vi "vetorcordist.vi"(9 "Parâmetros 2":T2={"Azul Max EV3 Cor"=17, "Azul Min EV3 Cor"=0, "Verde Max EV3 Cor"=6, "Verde Min EV3 Cor"=0, "Vermelho Max Ev3 Cor"=0, "Vermelho Min EV3 Cor"=0, "Chão EV3 Cor"=0.0, "Branco Max EV3 Cor"=0.0, "Branco Min EV3 Cor"=0.0, "Preto Max EV3 Cor"=0.0, "Preto Min EV3 Cor"=0.0, "Distância Tubulação"=0.0, "Distância Frontal"=0.0, "Amarelo Max EV3 Cor"=0.0, "Amarelo Min EV3 Cor"=0.0, "Distância Lateral"=0.0, "90°"=0.0, "180°"=0.0, "Seguidor de Linha"=0.0}, 11 "NXT/EV3 2":T1) -> (0 "dist perc":dbl, 3 "NXT/EV3 13":T1, 8 "cod cor":dbl format="%#_13g")   [LabVIEW 2016]
uses:
  <vilib>/NXT/Subs/LVHSConnector.ctl
  <vilib>/NXT/LegoClasses/BrickReference/BrickReference.lvclass
  <vilib>/NXT/Block Support/NXT_InputPort.ctl
  <vilib>/NXT/Block Support/NXT_OutputPort.ctl
  <vilib>/NXT/Dual Mode Library/Sensors/EV3_Gyro_Reset.vi
  <vilib>/NXT/Dual Mode Library/Motors/ResetMotor.vi
  <vilib>/NXT/Dual Mode Library/Sensors/EV3_Gyro_Angle.vi
  <vilib>/NXT/NXTIO Xnodes/NXTIONodeSubVIs/NXTStopMotors.vi
  <vilib>/NXT/Dual Mode Library/Motors/Rotation.vi
  <vilib>/NXT/NXTIO Xnodes/AddressXNode/NXTIOAddress.xnode
  <vilib>/NXT/NXTIO Xnodes/NXTIOXNode/NXTIO.xnode
panel:
  # "Sensor EV3 Cor"
  # "Sensor Ultrassônico"
  # "Sensor Giroscópio"
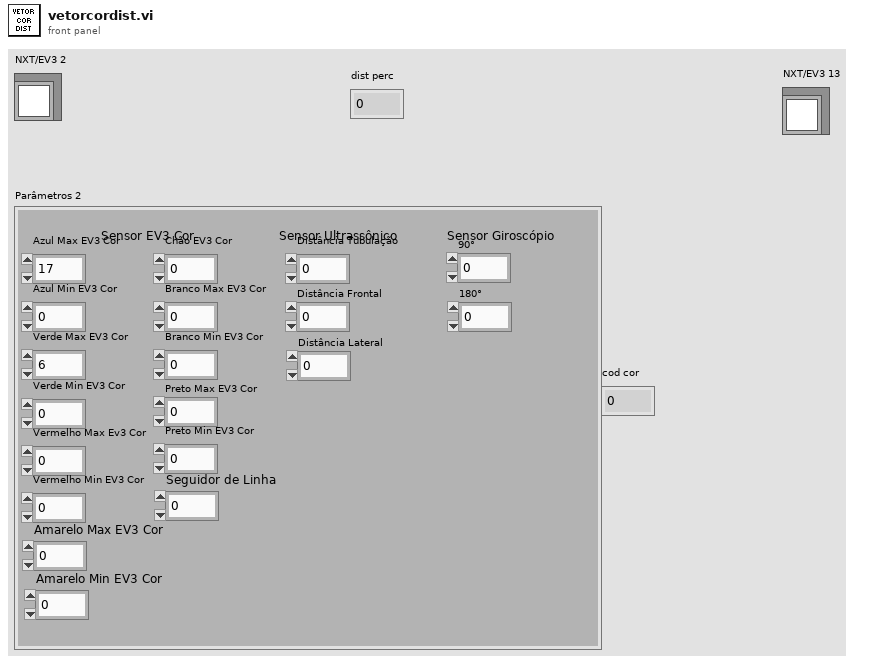
[diagram p1: front panel]
types:
  T1 = typedef "LVHSConnector.ctl" = refnum<class "BrickReference.lvclass">
  T2 = cluster{"Azul Max EV3 Cor":i32, "Azul Min EV3 Cor":i32, "Verde Max EV3 Cor":i32, "Verde Min EV3 Cor":i32, "Vermelho Max Ev3 Cor":i32, "Vermelho Min EV3 Cor":i32, "Chão EV3 Cor":sgl, "Branco Max EV3 Cor":sgl, "Branco Min EV3 Cor":sgl, "Preto Max EV3 Cor":sgl, "Preto Min EV3 Cor":sgl, "Distância Tubulação":sgl, "Distância Frontal":sgl, "Amarelo Max EV3 Cor":dbl, "Amarelo Min EV3 Cor":dbl, "Distância Lateral":sgl, "90°":sgl, "180°":sgl, "Seguidor de Linha":dbl}
  T3 = typedef "NXT_OutputPort.ctl" = u8
  T4 = typedef "NXT_InputPort.ctl" = u32
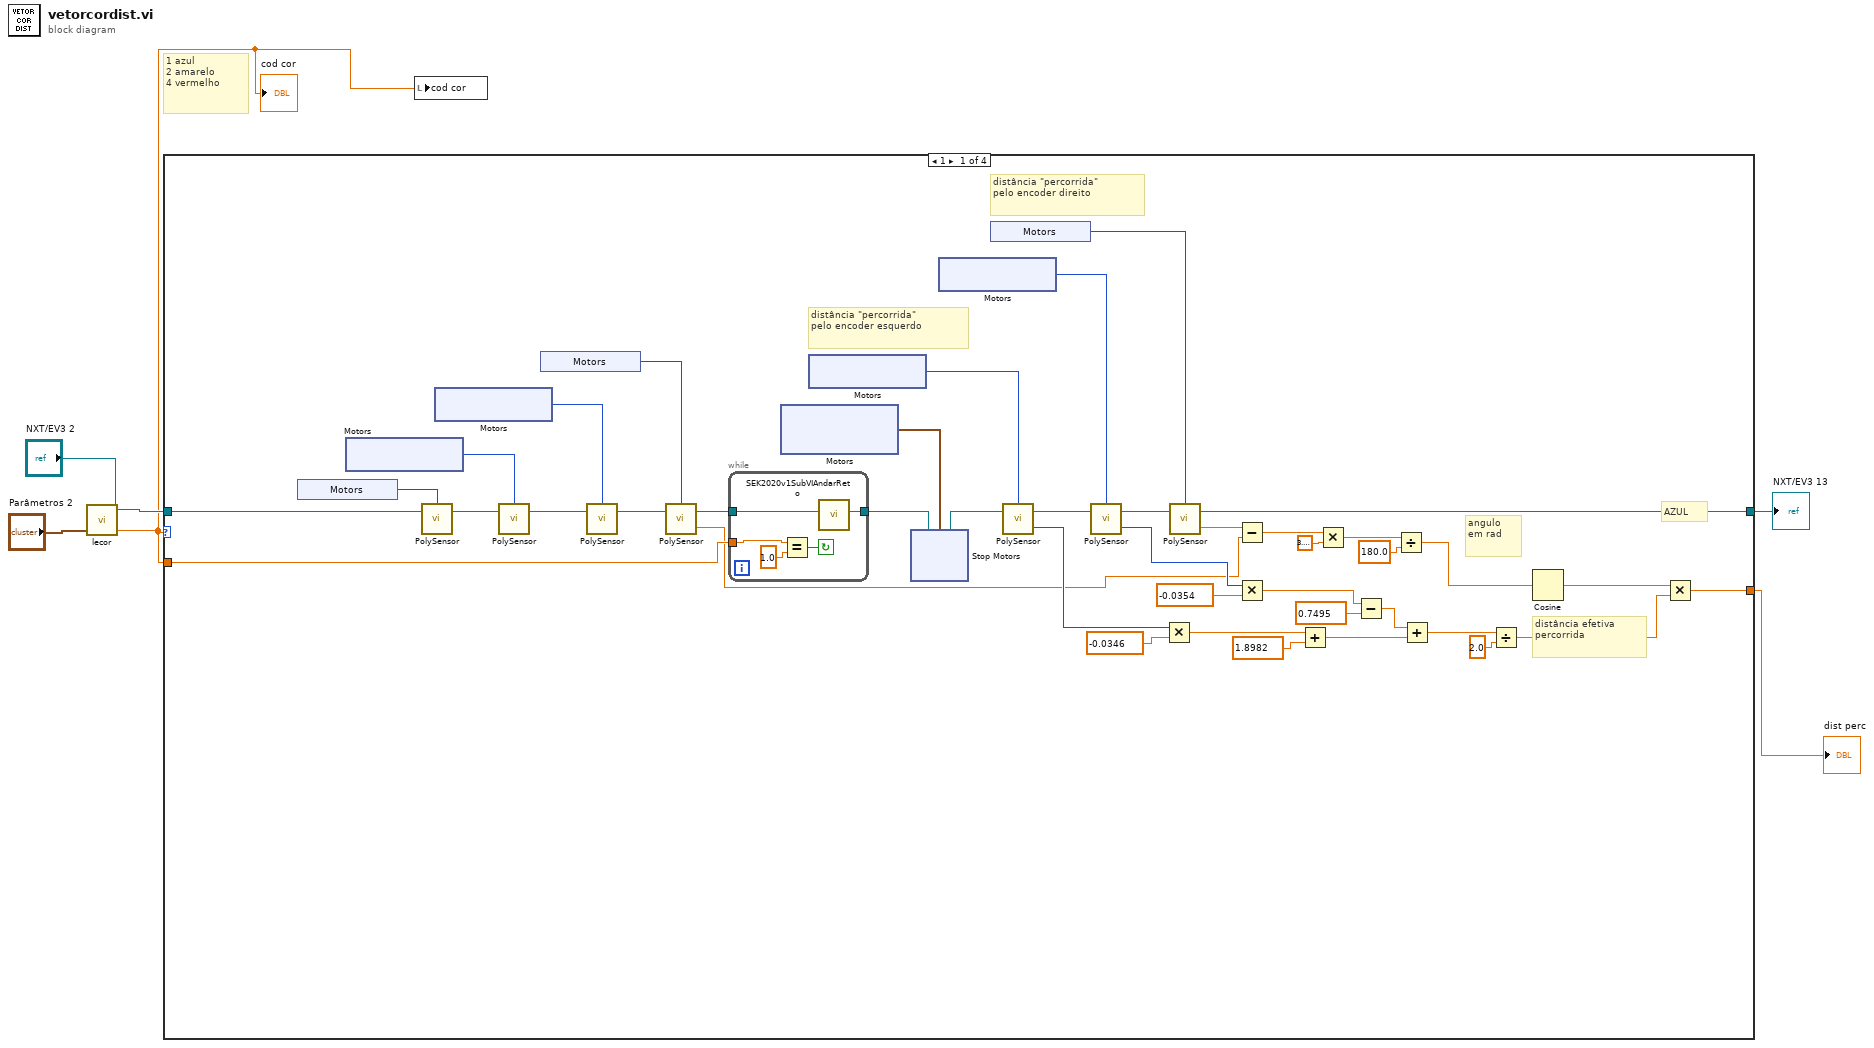
[diagram p0: block diagram]
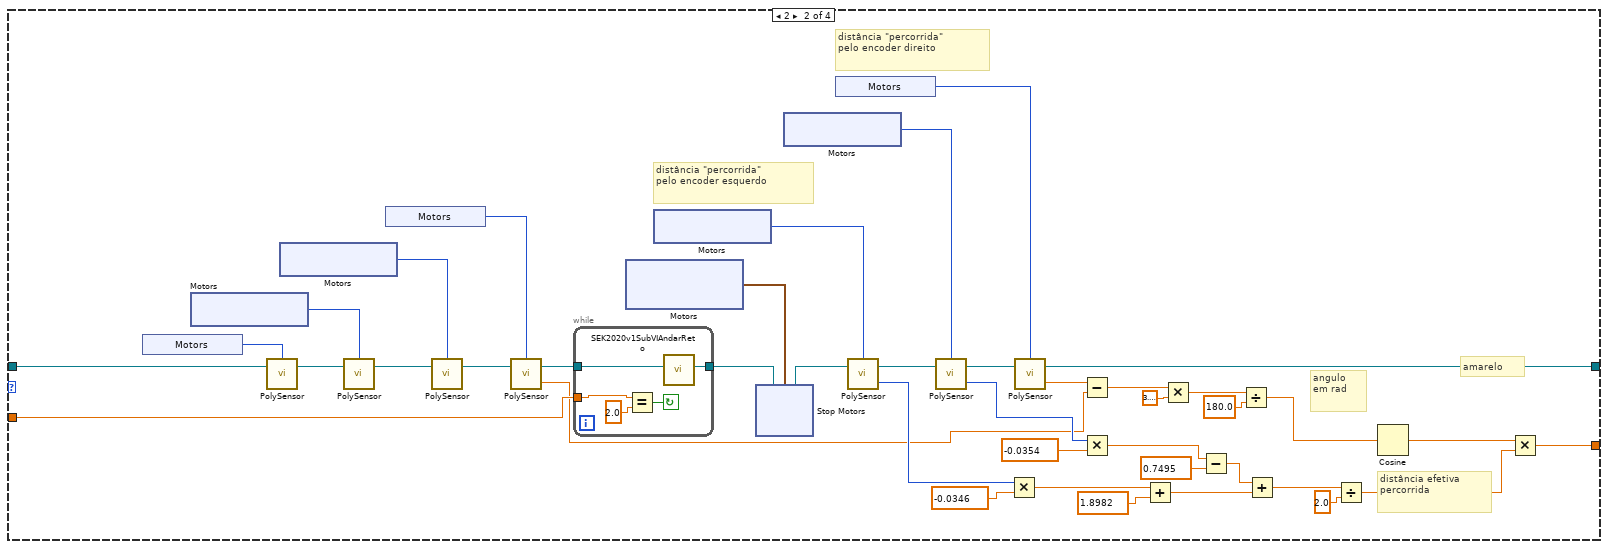
[diagram p2: hidden frame]
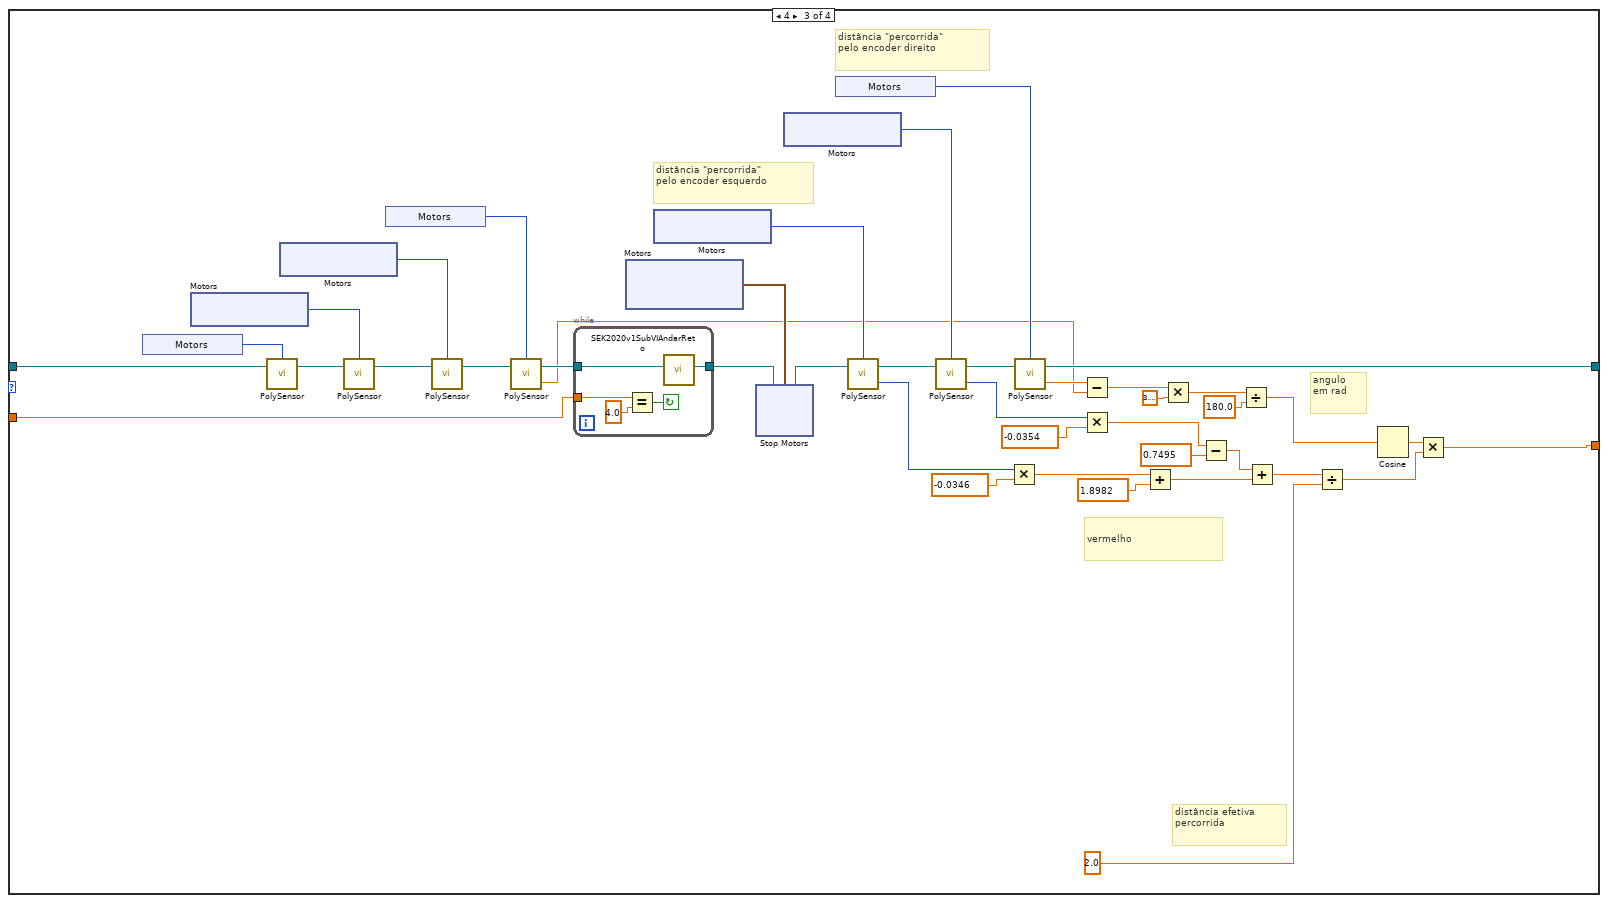
[diagram p3: hidden frame]
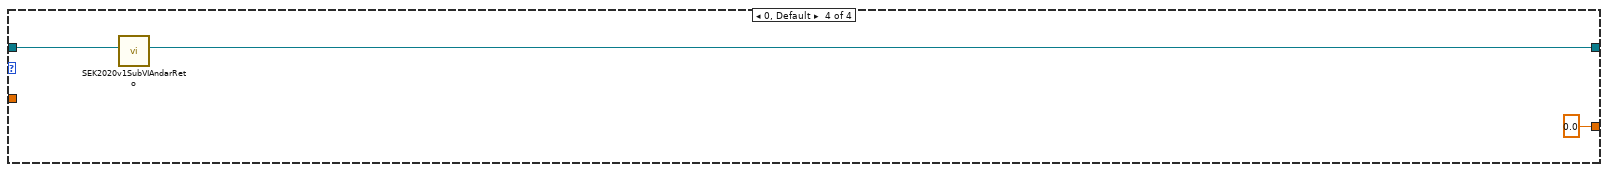
[diagram p4: hidden frame]
diagram:
  # "1 azul\n2 amarelo\n4 vermelho"
  n1 = call "lecor.vi"("Parâmetros 2"="Parâmetros 2", "NXT/EV3"="NXT/EV3 2") -> ("cor"=w1:dbl, "NXT/EV3 2"=w4:T1)  [unwired: 2 in]
  "cod cor" <- w1
  n2 = case shown="1" w1 {
    tunnel: w4 -> [w12 w71 w130 w186]
    tunnel: [w47 w106 w165 w185] -> w3
    tunnel: [w46 w105 w164 0.0] -> w2
    tunnel: w1 -> [w11 w70 w129 _]
    frame 1 {
      # "AZUL"
      # "angulo \nem rad"
      # "distância efetiva\npercorrida"
      # "distância \"percorrida\" \npelo encoder direito"
      # "distância \"percorrida\" \npelo encoder esquerdo"
      n3 = xnode "Motors"() -> ("Sensor"=w16:T4)
      n4 = xnode "Motors"() -> ("Motor"=w18:T3)
      n5 = call-poly <vilib>:"PolySensor.vi"("NXT/EV3"=w12, "Port (Port 1)"=w16) -> ("NXT/EV3"=w15:T1)  [unwired: 2 in]
      n6 = xnode "Motors"() -> ("Motor"=w13:T3)
      n7 = call-poly <vilib>:"PolySensor.vi"("NXT/EV3"=w15, "Port (All Ports)"=w18) -> ("NXT/EV3"=w17:T1)  [unwired: 2 in]
      n8 = xnode "Motors"() -> ("Sensor"=w10:T4)
      n9 = call-poly <vilib>:"PolySensor.vi"("NXT/EV3"=w17, "Port (All Ports)"=w13) -> ("NXT/EV3"=w9:T1)  [unwired: 2 in]
      n10 = call-poly <vilib>:"PolySensor.vi"("NXT/EV3"=w9, "Port (Port 1)"=w10) -> ("Degrees"=w7:sgl, "NXT/EV3"=w8:T1)  [unwired: 1 in]
      n11 = while {
        tunnel: [w53] -> w14
        tunnel: w11 -> [w50]
        tunnel: w8 -> [w49]
        stop <- w51 continue-if-true
        n12 = Equal?(x=w50, y=1.0) -> (x = y?=w51:bool)
        n13 = call "SEK2020v1SubVIAndarReto.vi"("NXT/EV3"=w49) -> ("NXT/EV3 2"=w53:T1)  [unwired: 9 in]
      }
      n14 = xnode "Motors"() -> ("Motor"=w25:cluster{"Port":T3, "Port":T3})
      n15 = xnode "Motors"() -> ("Motor"=w43:T3)
      n16 = xnode "Stop Motors"("Motors"=w25, "NXT/EV3"=w14) -> ("NXT/EV3"=w26:T1)
      n17 = xnode "Motors"() -> ("Motor"=w42:T3)
      n18 = xnode "Motors"() -> ("Sensor"=w45:T4)
      n19 = call-poly <vilib>:"PolySensor.vi"("NXT/EV3"=w26, "Port (Port A)"=w43) -> ("Angle of Rotation"=w40:i32, "NXT/EV3"=w41:T1)  [unwired: 1 in]
      n20 = call-poly <vilib>:"PolySensor.vi"("NXT/EV3"=w41, "Port (Port A)"=w42) -> ("Angle of Rotation"=w36:i32, "NXT/EV3"=w29:T1)  [unwired: 1 in]
      n21 = Multiply(x=w40, y=-0.0346) -> (x*y=w38:dbl)
      n22 = call-poly <vilib>:"PolySensor.vi"("NXT/EV3"=w29, "Port (Port 1)"=w45) -> ("Degrees"=w44:sgl, "NXT/EV3"=w47:T1)  [unwired: 1 in]
      n23 = Subtract(x=w44, y=w7) -> (x-y=w23:sgl)
      n24 = Multiply(x=w36, y=-0.0354) -> (x*y=w34:dbl)
      n25 = Add(x=w38, y=1.8982) -> (x+y=w28:dbl)
      n26 = Multiply(x=w23, y=3.141592653589793) -> (x*y=w21:dbl)
      n27 = Subtract(x=w34, y=0.7495) -> (x-y=w27:dbl)
      n28 = Divide(x=w21, y=180.0) -> (x/y=w19:dbl)
      n29 = Add(x=w27, y=w28) -> (x+y=w32:dbl)
      n30 = Divide(x=w32, y=2.0) -> (x/y=w30:dbl)
      n31 = Cosine(x=w19) -> (cos(x)=w24:dbl)
      n32 = Multiply(x=w24, y=w30) -> (x*y=w46:dbl)
    }
    frame 2 {
      # "amarelo"
      # "angulo \nem rad"
      # "distância efetiva\npercorrida"
      # "distância \"percorrida\" \npelo encoder direito"
      # "distância \"percorrida\" \npelo encoder esquerdo"
      n33 = xnode "Motors"() -> ("Sensor"=w75:T4)
      n34 = xnode "Motors"() -> ("Motor"=w77:T3)
      n35 = call-poly <vilib>:"PolySensor.vi"("NXT/EV3"=w71, "Port (Port 1)"=w75) -> ("NXT/EV3"=w74:T1)  [unwired: 2 in]
      n36 = xnode "Motors"() -> ("Motor"=w72:T3)
      n37 = call-poly <vilib>:"PolySensor.vi"("NXT/EV3"=w74, "Port (All Ports)"=w77) -> ("NXT/EV3"=w76:T1)  [unwired: 2 in]
      n38 = xnode "Motors"() -> ("Sensor"=w69:T4)
      n39 = call-poly <vilib>:"PolySensor.vi"("NXT/EV3"=w76, "Port (All Ports)"=w72) -> ("NXT/EV3"=w67:T1)  [unwired: 2 in]
      n40 = call-poly <vilib>:"PolySensor.vi"("NXT/EV3"=w67, "Port (Port 1)"=w69) -> ("Degrees"=w68:sgl, "NXT/EV3"=w66:T1)  [unwired: 1 in]
      n41 = while {
        tunnel: w66 -> [w112]
        tunnel: [w111] -> w73
        tunnel: w70 -> [w108]
        stop <- w109 continue-if-true
        n42 = Equal?(x=w108, y=2.0) -> (x = y?=w109:bool)
        n43 = call "SEK2020v1SubVIAndarReto.vi"("NXT/EV3"=w112) -> ("NXT/EV3 2"=w111:T1)  [unwired: 9 in]
      }
      n44 = xnode "Motors"() -> ("Motor"=w84:cluster{"Port":T3, "Port":T3})
      n45 = xnode "Motors"() -> ("Motor"=w102:T3)
      n46 = xnode "Stop Motors"("Motors"=w84, "NXT/EV3"=w73) -> ("NXT/EV3"=w85:T1)
      n47 = xnode "Motors"() -> ("Motor"=w101:T3)
      n48 = xnode "Motors"() -> ("Sensor"=w104:T4)
      n49 = call-poly <vilib>:"PolySensor.vi"("NXT/EV3"=w85, "Port (Port A)"=w102) -> ("Angle of Rotation"=w99:i32, "NXT/EV3"=w100:T1)  [unwired: 1 in]
      n50 = call-poly <vilib>:"PolySensor.vi"("NXT/EV3"=w100, "Port (Port A)"=w101) -> ("Angle of Rotation"=w95:i32, "NXT/EV3"=w88:T1)  [unwired: 1 in]
      n51 = Multiply(x=w99, y=-0.0346) -> (x*y=w97:dbl)
      n52 = call-poly <vilib>:"PolySensor.vi"("NXT/EV3"=w88, "Port (Port 1)"=w104) -> ("Degrees"=w103:sgl, "NXT/EV3"=w106:T1)  [unwired: 1 in]
      n53 = Subtract(x=w103, y=w68) -> (x-y=w82:sgl)
      n54 = Multiply(x=w95, y=-0.0354) -> (x*y=w93:dbl)
      n55 = Add(x=w97, y=1.8982) -> (x+y=w87:dbl)
      n56 = Multiply(x=w82, y=3.141592653589793) -> (x*y=w80:dbl)
      n57 = Subtract(x=w93, y=0.7495) -> (x-y=w86:dbl)
      n58 = Divide(x=w80, y=180.0) -> (x/y=w78:dbl)
      n59 = Add(x=w86, y=w87) -> (x+y=w91:dbl)
      n60 = Divide(x=w91, y=2.0) -> (x/y=w89:dbl)
      n61 = Cosine(x=w78) -> (cos(x)=w83:dbl)
      n62 = Multiply(x=w83, y=w89) -> (x*y=w105:dbl)
    }
    frame 4 {
      # "vermelho"
      # "angulo \nem rad"
      # "distância efetiva\npercorrida"
      # "distância \"percorrida\" \npelo encoder direito"
      # "distância \"percorrida\" \npelo encoder esquerdo"
      n63 = xnode "Motors"() -> ("Sensor"=w134:T4)
      n64 = xnode "Motors"() -> ("Motor"=w136:T3)
      n65 = call-poly <vilib>:"PolySensor.vi"("NXT/EV3"=w130, "Port (Port 1)"=w134) -> ("NXT/EV3"=w133:T1)  [unwired: 2 in]
      n66 = xnode "Motors"() -> ("Motor"=w131:T3)
      n67 = call-poly <vilib>:"PolySensor.vi"("NXT/EV3"=w133, "Port (All Ports)"=w136) -> ("NXT/EV3"=w135:T1)  [unwired: 2 in]
      n68 = xnode "Motors"() -> ("Sensor"=w128:T4)
      n69 = call-poly <vilib>:"PolySensor.vi"("NXT/EV3"=w135, "Port (All Ports)"=w131) -> ("NXT/EV3"=w127:T1)  [unwired: 2 in]
      n70 = call-poly <vilib>:"PolySensor.vi"("NXT/EV3"=w127, "Port (Port 1)"=w128) -> ("Degrees"=w125:sgl, "NXT/EV3"=w126:T1)  [unwired: 1 in]
      n71 = while {
        tunnel: [w171] -> w132
        tunnel: w129 -> [w168]
        tunnel: w126 -> [w167]
        stop <- w169 continue-if-true
        n72 = Equal?(x=w168, y=4.0) -> (x = y?=w169:bool)
        n73 = call "SEK2020v1SubVIAndarReto.vi"("NXT/EV3"=w167) -> ("NXT/EV3 2"=w171:T1)  [unwired: 9 in]
      }
      n74 = xnode "Motors"() -> ("Motor"=w143:cluster{"Port":T3, "Port":T3})
      n75 = xnode "Motors"() -> ("Motor"=w161:T3)
      n76 = xnode "Stop Motors"("Motors"=w143, "NXT/EV3"=w132) -> ("NXT/EV3"=w144:T1)
      n77 = xnode "Motors"() -> ("Motor"=w160:T3)
      n78 = xnode "Motors"() -> ("Sensor"=w163:T4)
      n79 = call-poly <vilib>:"PolySensor.vi"("NXT/EV3"=w144, "Port (Port A)"=w161) -> ("Angle of Rotation"=w158:i32, "NXT/EV3"=w159:T1)  [unwired: 1 in]
      n80 = call-poly <vilib>:"PolySensor.vi"("NXT/EV3"=w159, "Port (Port A)"=w160) -> ("Angle of Rotation"=w154:i32, "NXT/EV3"=w147:T1)  [unwired: 1 in]
      n81 = Multiply(x=w158, y=-0.0346) -> (x*y=w156:dbl)
      n82 = call-poly <vilib>:"PolySensor.vi"("NXT/EV3"=w147, "Port (Port 1)"=w163) -> ("Degrees"=w162:sgl, "NXT/EV3"=w165:T1)  [unwired: 1 in]
      n83 = Subtract(x=w162, y=w125) -> (x-y=w141:sgl)
      n84 = Multiply(x=w154, y=-0.0354) -> (x*y=w152:dbl)
      n85 = Add(x=w156, y=1.8982) -> (x+y=w146:dbl)
      n86 = Multiply(x=w141, y=3.141592653589793) -> (x*y=w139:dbl)
      n87 = Subtract(x=w152, y=0.7495) -> (x-y=w145:dbl)
      n88 = Divide(x=w139, y=180.0) -> (x/y=w137:dbl)
      n89 = Add(x=w145, y=w146) -> (x+y=w150:dbl)
      n90 = Divide(x=w150, y=2.0) -> (x/y=w148:dbl)
      n91 = Cosine(x=w137) -> (cos(x)=w142:dbl)
      n92 = Multiply(x=w142, y=w148) -> (x*y=w164:dbl)
    }
    frame 0, Default {
      n93 = call "SEK2020v1SubVIAndarReto.vi"("NXT/EV3"=w186) -> ("NXT/EV3 2"=w185:T1)  [unwired: 9 in]
    }
  }
  "NXT/EV3 13" <- w3
  "dist perc" <- w2
  n94 = local write "cod cor"(w1) -> ()
